vi "Note Dialog.vi"(8 "error in (no error)":errorcluster) -> (0 "error out":errorcluster, 1 "Note":string, 2 "OK":bool)   [LabVIEW 2021, in "CSV Log.lvlib"]
uses:
  CSV Log.lvlib
panel:
  in  "Cancel Button":bool
  in  "OK Button":bool
  in  "Enter Note":string
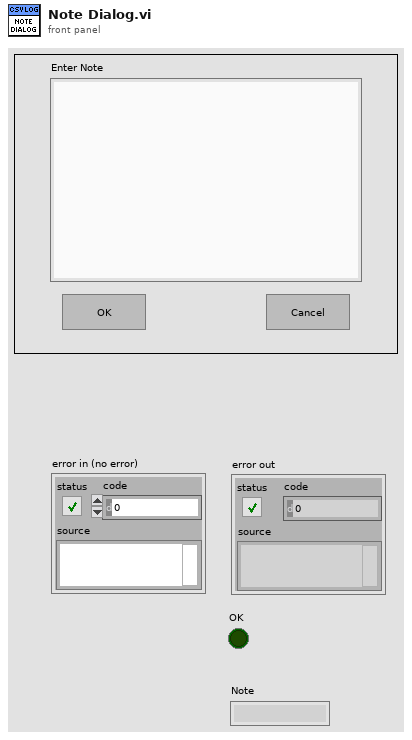
[diagram p1: front panel]
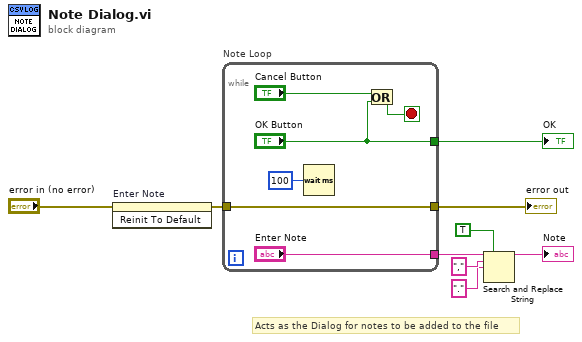
[diagram p0: block diagram]
diagram:
  # "Acts as the Dialog for notes to be added to the file"
  n1 = invoke on="Enter Note" class="Str" method="Reinit To Default"(error in="error in (no error)") -> (error out=w6:errorcluster)  [unwired: 2 in, 2 out]
  n2 = while "Note Loop" {
    tunnel: [w15] -> w9
    tunnel: w6 -> [w15]
    tunnel: ["OK Button"] -> w8
    tunnel: ["Enter Note"] -> w5
    stop <- w13 stop-if-true
    n3 = Wait (ms)(milliseconds to wait=u32 100) -> ()  [unwired: 1 out]
    n4 = Or(x="Cancel Button", y="OK Button") -> (x .or. y?=w13:bool)
  }
  "error out" <- w9
  "OK" <- w8
  n5 = Search and Replace String(replace all?=TRUE ("replace all? (F)"), input string=w5, search string=",", replace string="." ("replace string (\"\")")) -> (result string=→"Note":string)  [unwired: 4 in, 3 out]
